vi "MedianFilter_New.vi"(11 "Samples":i32) -> (3 "MEDIAN_FILTER":T1 {"ValueBuffer" format="%13.5g"})   [LabVIEW 2019, in "Trajectory_Library.lvlib"]
doc: "Creates a new MedianFilter data cluster.\n\nThis implements a moving-window median filter. Useful for reducing measurement noise, especially with processes that generate occasional, extreme outliers (such as values from vision processing, LIDAR, or ultrasonic sensors).\n\nInputs:\n - samples -- The number of samples in the moving window.\n\nOutputs:\n - Median Filter -- Median filter data structure"
uses:
  Trajectory_Library.lvlib
  TypeDef/MEDIAN_FILTER.ctl
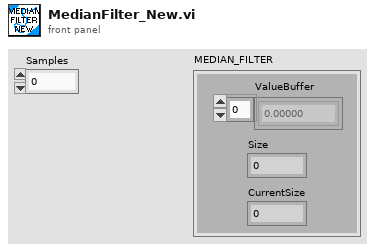
[diagram p1: front panel]
types:
  T1 = typedef "Trajectory_Library.lvlib/MEDIAN_FILTER.ctl" = cluster{"ValueBuffer":dbl[], "Size":i32, "CurrentSize":i32}
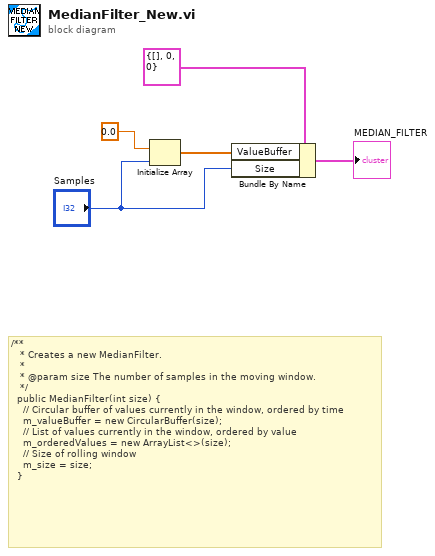
[diagram p0: block diagram]
diagram:
  # "/**\n   * Creates a new MedianFilter.\n   *\n   * @param size The number of samples in the moving window.\n   */\n  public MedianFilter(int size) {\n    // Circular buffer of values currently in the window, ordered by time\n    m_valueBuffer = new CircularBuffer(size);\n    // List of values currently in the window, ordered by value\n    m_orderedValues = new ArrayList<>(size);\n    // Size of rolling window\n    m_size = size;\n  }"
  n1 = Initialize Array(0.0 ("element"), "Samples") -> (w2:dbl[])
  n2 = Bundle By Name(cluster=T1 {"ValueBuffer"=[], "Size"=0, "CurrentSize"=0} ("MEDIAN_FILTER"), "ValueBuffer"=w2, "Size"="Samples") -> (→"MEDIAN_FILTER":T1)
